vi "Check Quit Conditions.vi"(8 "error in (no error)":errorcluster) -> (0 "error out":errorcluster, 2 "Quit?":bool)   [LabVIEW 2016, in "Hall Effect Library.lvlib"]
doc: "Returns Quit? = True if there is an error on error in or if the user sent an ABORT."
uses:
  Hall Effect Library.lvlib
  Global Variables/Communication.vi
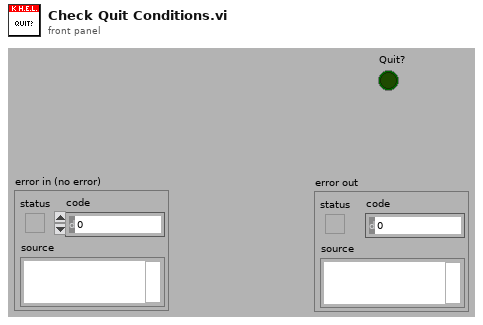
[diagram p1: front panel]
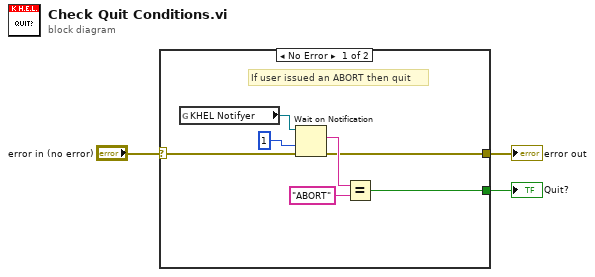
[diagram p0: block diagram]
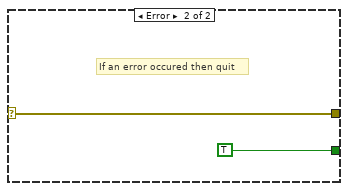
[diagram p2: hidden frame]
diagram:
  n1 = case shown="No Error" "error in (no error)" {
    selector: "error in (no error)" -> [w8 w12]
    tunnel: [w5 w12] -> w2
    tunnel: [w4 TRUE] -> w1
    frame No Error {
      # "If user issued an ABORT then quit"
      n2 = global read "Communication.vi" "KHEL Notifyer"() -> (w10:refnum<notifier>)
      n3 = Wait on Notification(notifier=w10, timeout in ms (-1)=1, error in (no error)=w8) -> (notification=w7:string, error out=w5:errorcluster)  [unwired: 3 out]
      n4 = Equal?(x=w7, y="ABORT") -> (x = y?=w4:bool)
    }
    frame Error {
      # "If an error occured then quit"
    }
  }
  "error out" <- w2
  "Quit?" <- w1
